vi "Temperature.vi"(8 "error in (no error)":errorcluster, 10 "Temperature unit":enum16{"C", "K", "F"}(ring), 11 "Sensor General Class in":refnum<class "Sensor General Class.lvclass">) -> (0 "error out":errorcluster, 2 "Temperature":sgl, 3 "Sensor General Class out":refnum<class "Sensor General Class.lvclass">)   [LabVIEW 2020, in "Sensor General Class.lvclass"]
uses:
  Sensor General Class.lvclass
  Data Enum.ctl
  Sensor General Class.lvclass/Sensor General Class.ctl
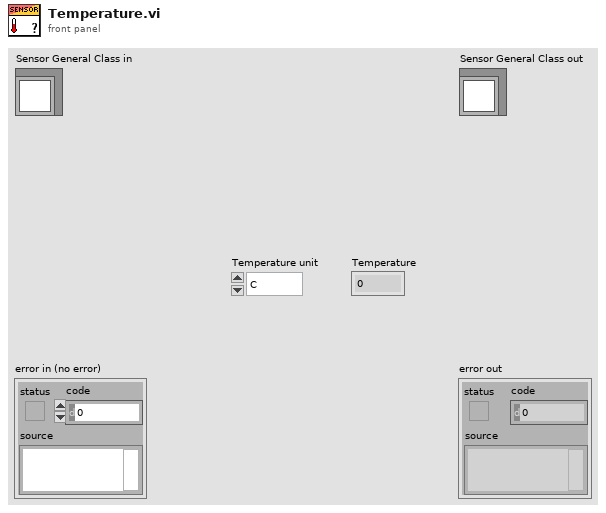
[diagram p1: front panel]
types:
  T1 = typedef "Sensor General Class.lvclass/Data Enum.ctl" = enum16{"p_bar", "p_MPa", "p_Pa", "p_kPa", "p_psi", "p_H/cm^2", "t_C", "t_K", "t_F", "rho_g/l", "rho_kg/m^3", "p20_bar", "related p20_bar", "p20_MPa", "related p20_MPa", "Tf_SF6", "Td_sf6", "tank Tf_SF6", "tank Td_SF6", "Tf_N2", "Td_N2", "tank Tf_N2", "tank Td_N2", "ppm_v SF6", "ppm_w SF6", "ppm_v N2", "ppm_w N2", "rH"}
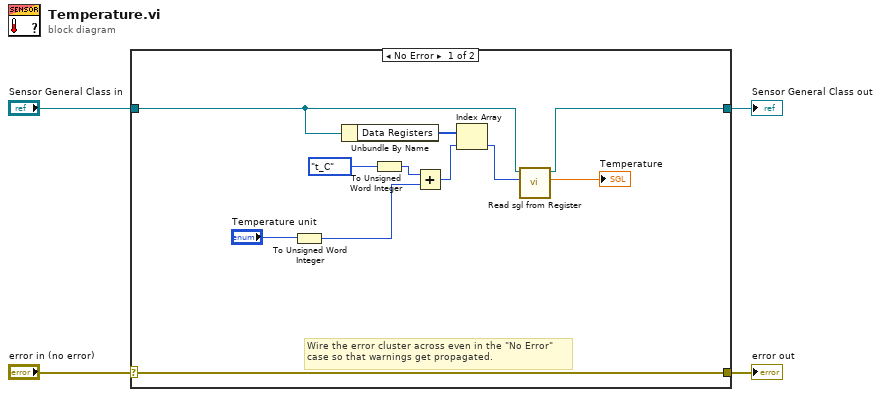
[diagram p0: block diagram]
diagram:
  n1 = case shown="No Error" "error in (no error)" {
    selector: "error in (no error)" -> [w15 w17]
    tunnel: [w15 w17] -> w3
    tunnel: [w9 w16] -> w1
    tunnel: "Sensor General Class in" -> [w8 w16]
    frame No Error {
      # "Wire the error cluster across even in the \"No Error\"\ncase so that warnings get propagated."
      n2 = To Unsigned Word Integer(number="Temperature unit") -> (unsigned 16bit integer=w11:u16)
      n3 = Unbundle By Name(w8) -> ("Data Registers"=w7:u16[])
      n4 = To Unsigned Word Integer(number=Data_Enum."t_C" ("Data Enum")) -> (unsigned 16bit integer=w12:u16)
      n5 = Add(x=w12, y=w11) -> (x+y=w6:u16)
      n6 = Index Array(array=w7, index=w6) -> (element=w5:u16)
      n7 = call-dynamic "Read sgl from Register.vi"("Start Register"=w5, "Sensor General Class in"=w8) -> ("Data"=→"Temperature":sgl, "Sensor General Class out"=w9:refnum<class "Sensor General Class.lvclass">)  [unwired: 7 in, 1 out]
    }
    frame Error {
    }
  }
  "error out" <- w3
  "Sensor General Class out" <- w1
